vi "Inventory-PayloadFromDB.vi"(8 "error in (no error)":errorcluster, 10 "JSON string":string, 11 "ERP-Inventory in":refnum<class "ERP-Inventory.lvclass">) -> (0 "error out":errorcluster, 3 "ERP-Inventory out":refnum<class "ERP-Inventory.lvclass">)   [LabVIEW 2013, in "ERP-Inventory.lvclass"]
uses:
  ERP-Inventory.lvclass
  ERP-Inventory.lvclass/ERP-Inventory.ctl
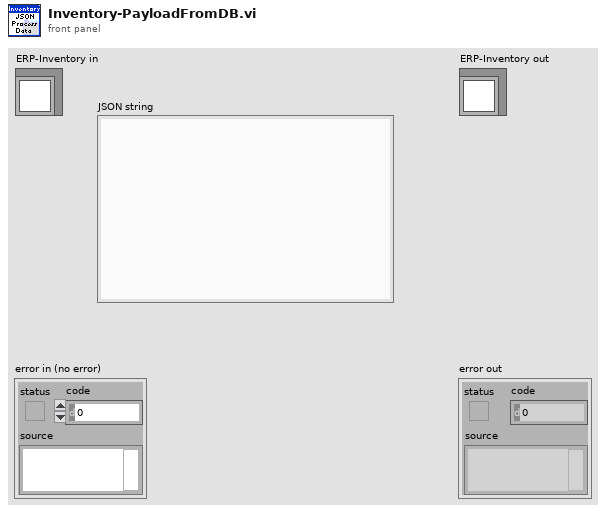
[diagram p1: front panel]
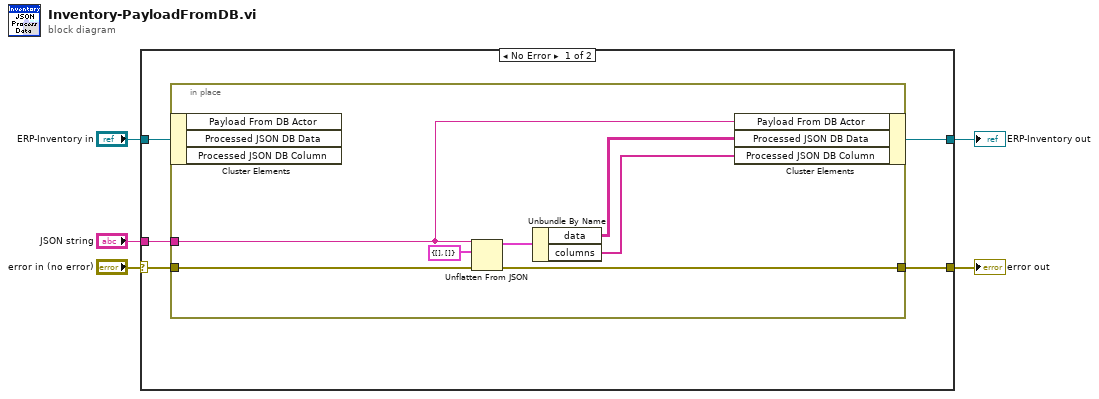
[diagram p0: block diagram]
diagram:
  n1 = case shown="No Error" "error in (no error)" {
    selector: "error in (no error)" -> [w8 w19]
    tunnel: [w7 w19] -> w4
    tunnel: [w9 w18] -> w2
    tunnel: "ERP-Inventory in" -> [w10 w18]
    tunnel: "JSON string" -> [w6 _]
    frame No Error {
      n2 = in-place {
        in-place-border: w8 -> [w13]
        in-place-border: [w12] -> w7
        in-place-border: w6 -> [w11]
        n3 = in-place-cluster #1(w10) -> ()  [unwired: 3 out]
        n4 = Unflatten From JSON(JSON string=w11, type and defaults=cluster{"data":string[][], "columns":string[]} {"data"=[], "columns"=[]}, error in (no error)=w13) -> (value=w17:cluster{"data":string[][], "columns":string[]}, error out=w12:errorcluster)  [unwired: 4 in]
        n5 = Unbundle By Name(w17) -> ("data"=w15:string[][], "columns"=w14:string[])
        n6 = in-place-cluster #1("Payload From DB Actor"=w11, "Processed JSON DB Data"=w15, "Processed JSON DB Column"=w14) -> (w9:refnum<class "ERP-Inventory.lvclass">)
      }
    }
    frame Error {
    }
  }
  "error out" <- w4
  "ERP-Inventory out" <- w2
